vi "uBroker_Core.vi"(10 "ActorCore Transport":refnum<class "uTransport_uActor.lvclass">, 11 "brokerage queue in":refnum<queue>) -> (3 "brokerage queue out":refnum<queue>)   [LabVIEW 2021, in "uFramework.lvlib" / "uBroker.lvclass"]
doc: "This is a helper loop for the actor core. It reduces dynamic dispatching in the brokerage functions as it avoid contiuous recalls of the EXEC method."
uses:
  uBroker.lvclass
  uBroker.lvclass/uBroker.ctl
  uClient_Subscriber/uClient_Subscriber.lvclass
  Bin/uData.lvlibp/uData.lvclass
  <vilib>/Utility/miscctls.llb/LVMapReplaceAction.ctl
  uClient_Publisher/uClient_Publisher.lvclass
  uSubscription/uSubscription.lvclass
  uMsg/uMsg.lvclass
  uTransport_uActor/uTransport_uActor.lvclass
  TypeDef_uBrokerTopic.ctl
panel:
  in  "Subscribers":set{refnum<class "uClient_Subscriber.lvclass">}(c389)
  in  "Topics":map{string, T1}(c390)
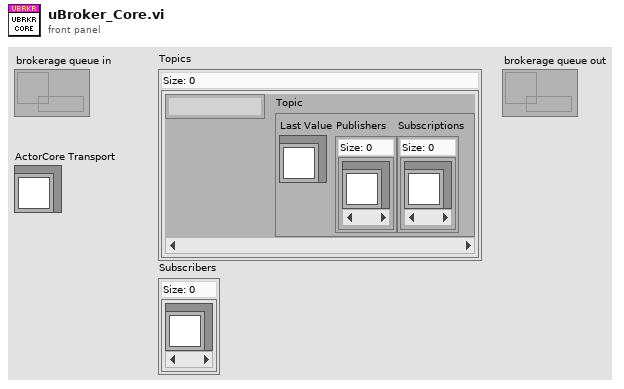
[diagram p1: front panel]
types:
  T1 = typedef "uFramework.lvlib/uBroker.lvclass/TypeDef_uBrokerTopic.ctl" = cluster{"Last Value":refnum<class "uMsg.lvclass">, "Publishers":set{refnum<class "uClient_Publisher.lvclass">}, "Subscriptions":set{refnum<class "uSubscription.lvclass">}}
  T2 = cluster{"Topics":map{string, T1}, "Subscribers":set{refnum<class "uClient_Subscriber.lvclass">}}
  T3 = typedef "LVMapReplaceAction.ctl" = enum32{"Modify Entry only if found", "Add or Modify Entry", "Delete Entry"}
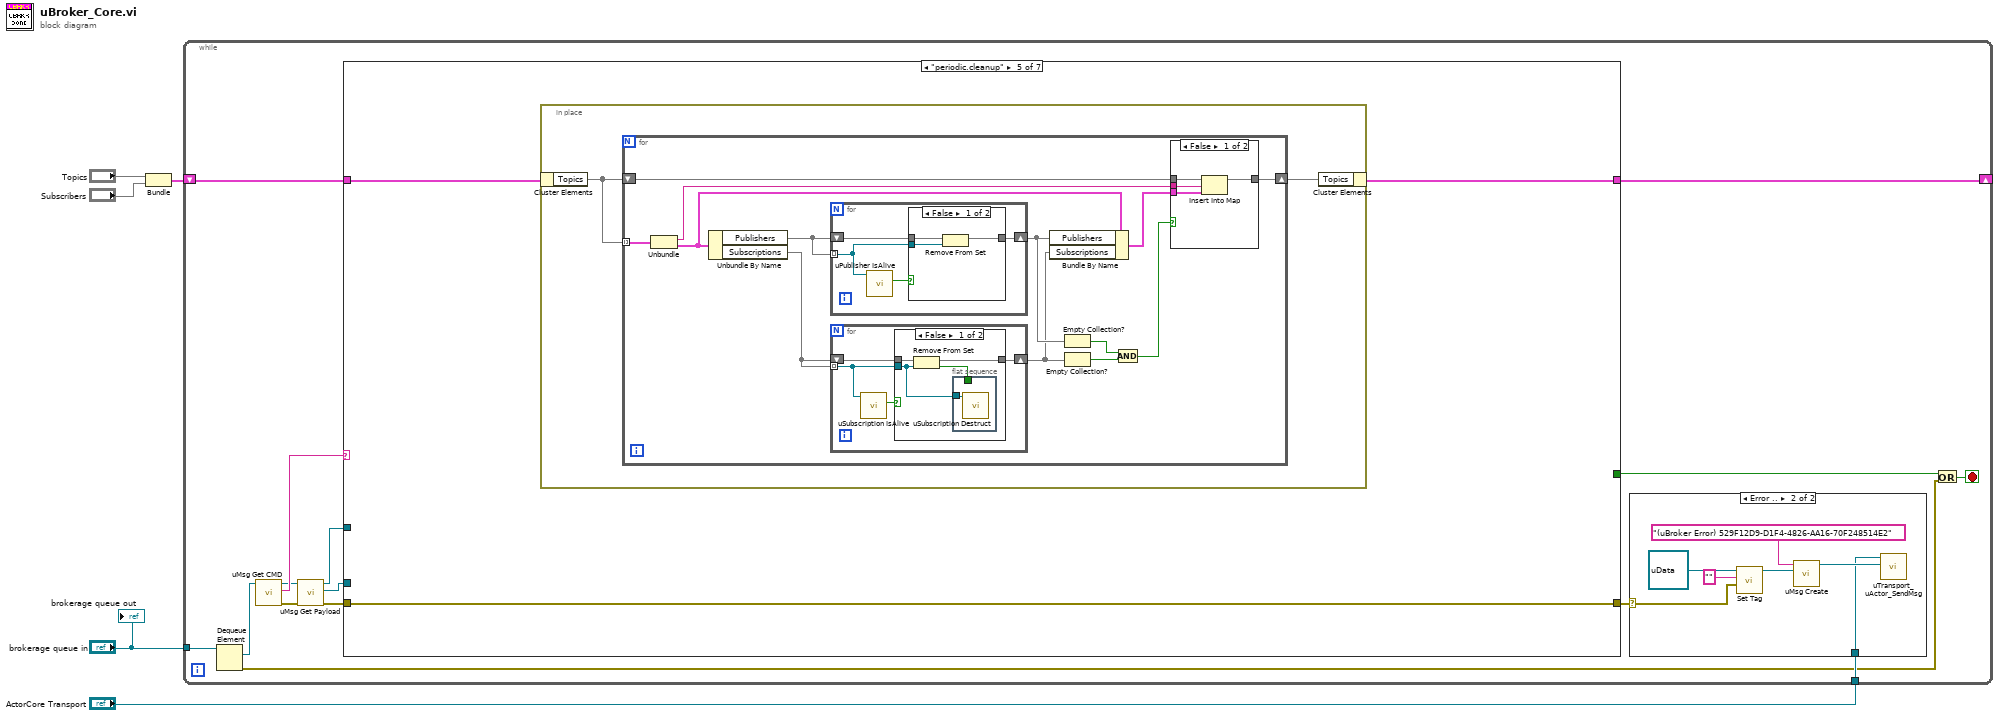
[diagram p0: block diagram]
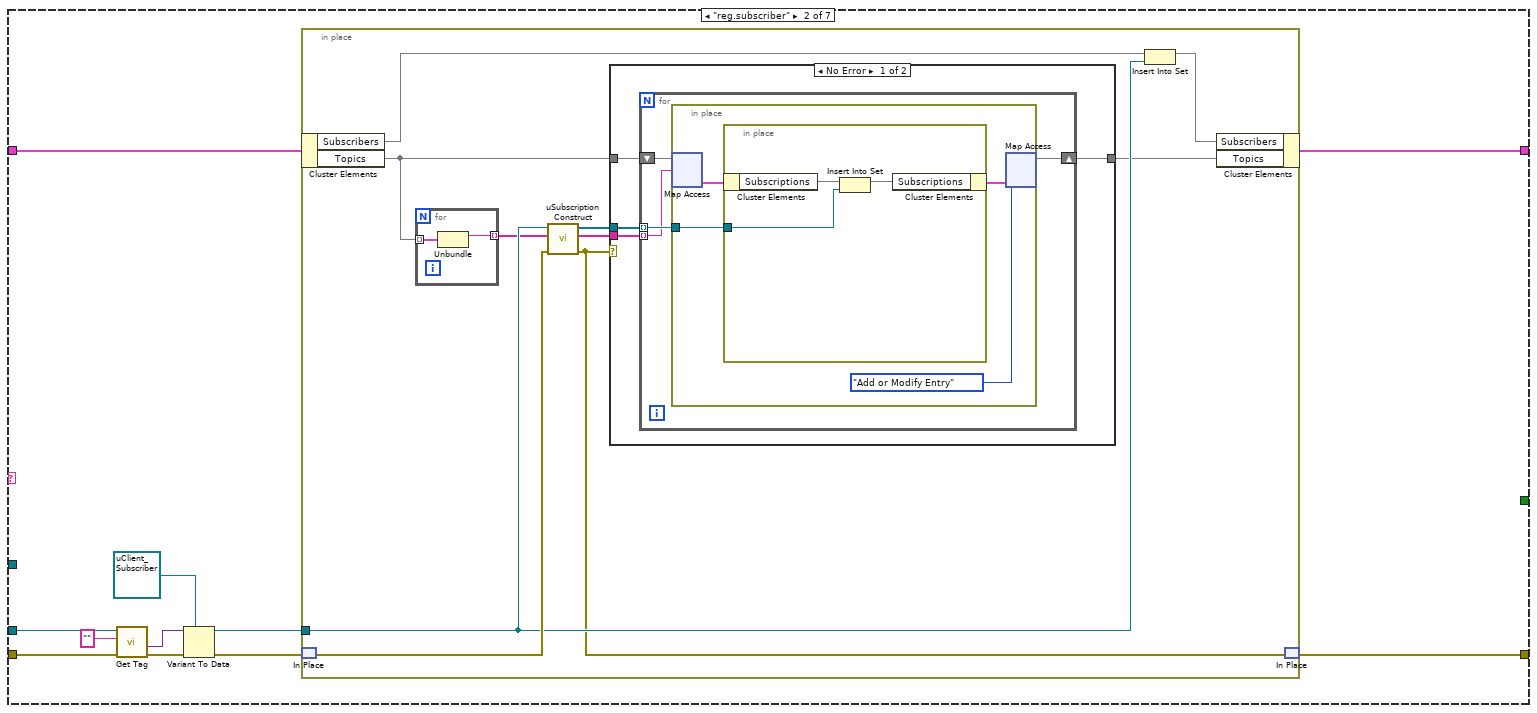
[diagram p4: hidden frame]
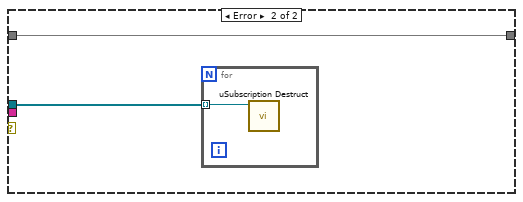
[diagram p5: hidden frame]
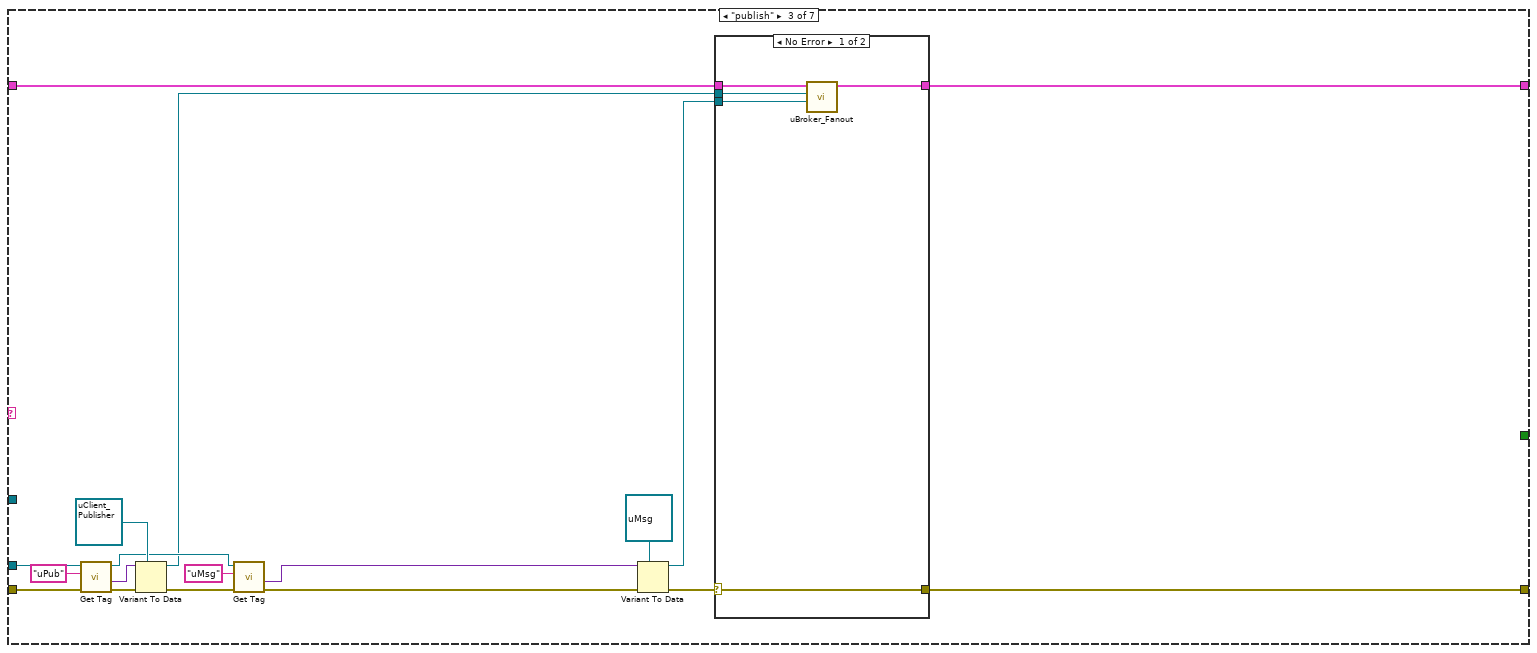
[diagram p6: hidden frame]
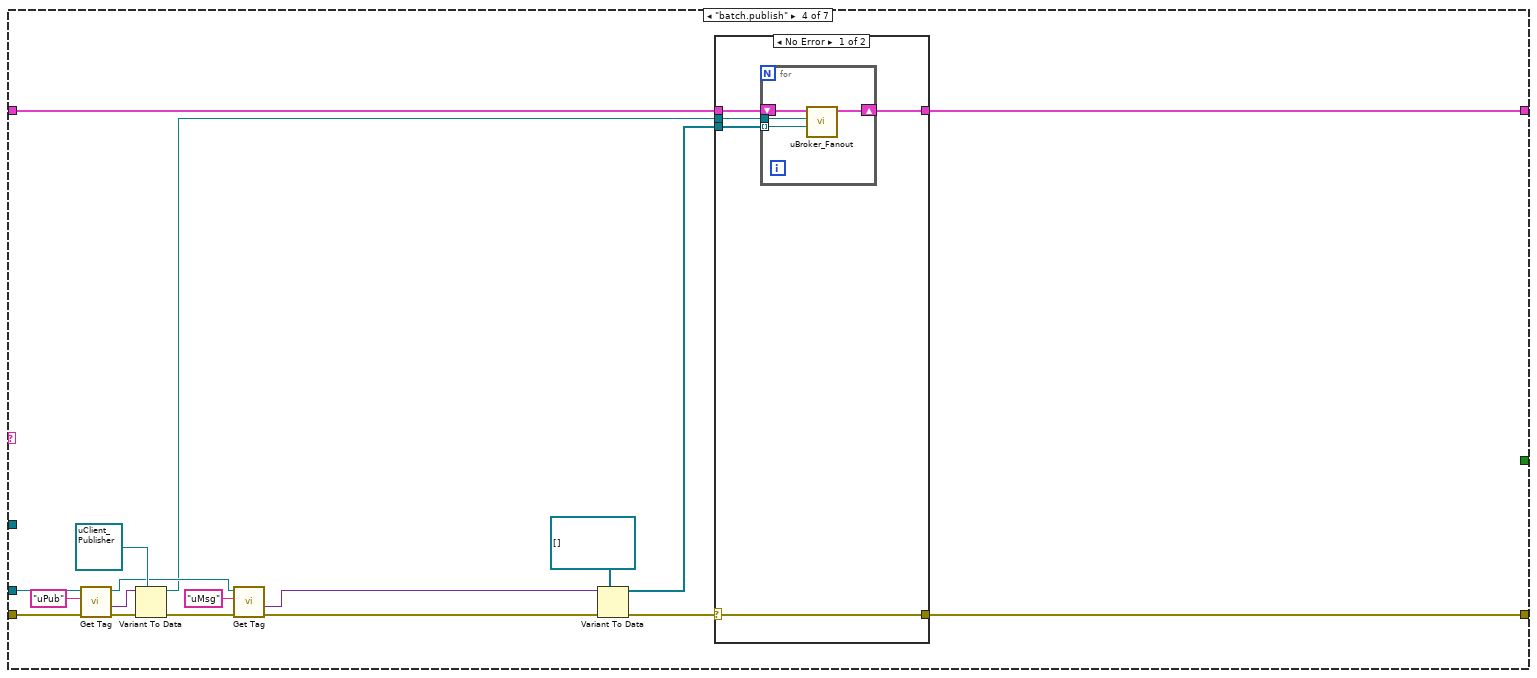
[diagram p8: hidden frame]
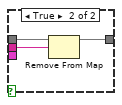
[diagram p10: hidden frame]
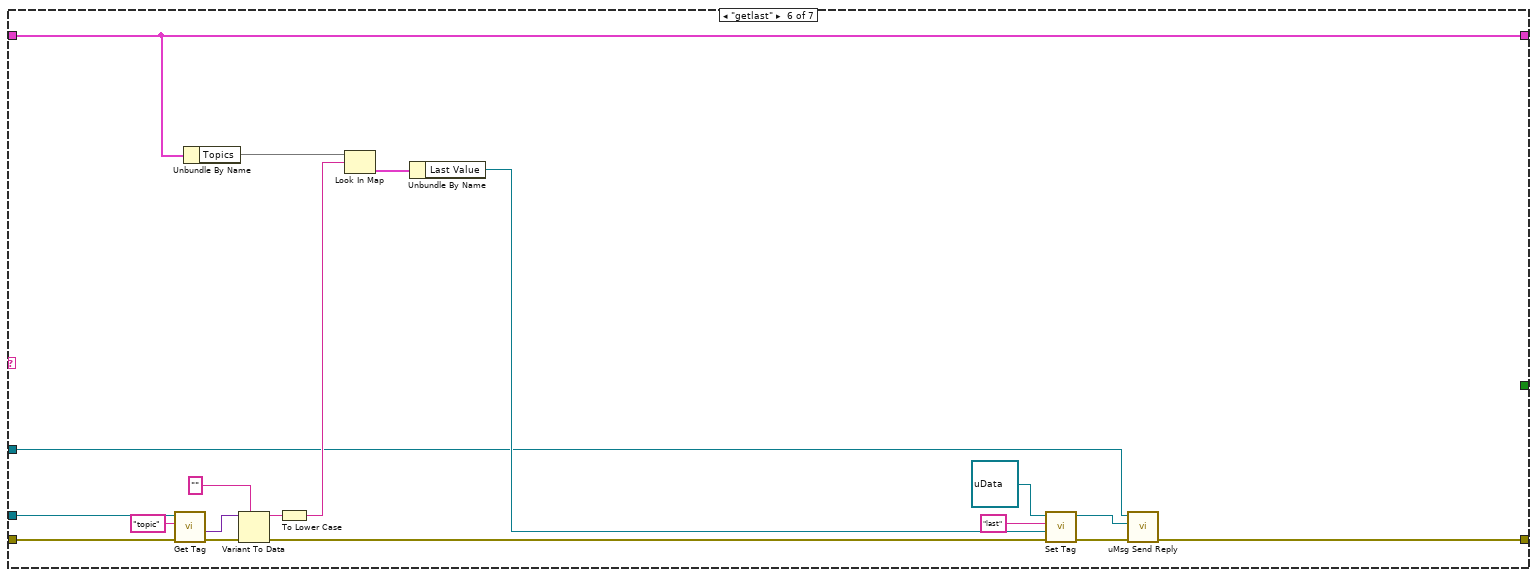
[diagram p13: hidden frame]
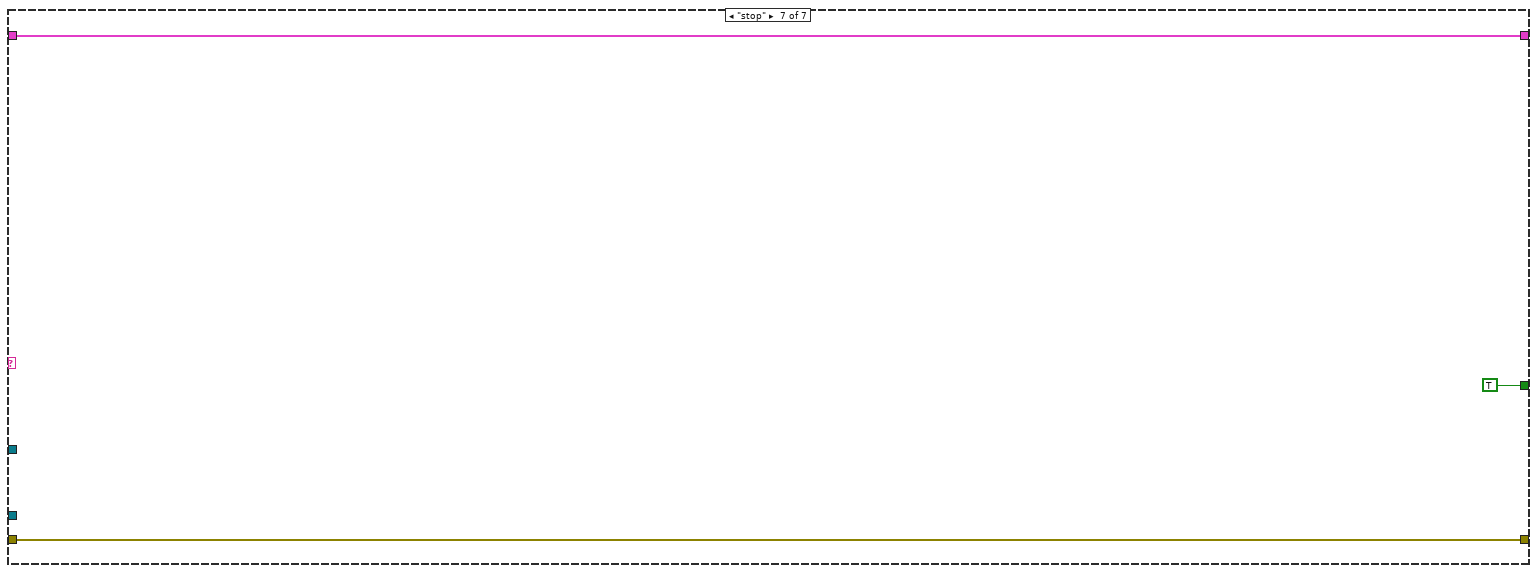
[diagram p14: hidden frame]
diagram:
  n1 = Bundle("Topics"="Topics", "Subscribers"="Subscribers") -> (w3:T2)  [unwired: 1 in]
  n2 = while {
    tunnel: "brokerage queue in" -> [w20]
    tunnel: "ActorCore Transport" -> [w16]
    shift-right: [w14] -> _
    shift-left: w3 -> [w15]
    stop <- w7 stop-if-true
    n3 = Dequeue Element(queue=w20) -> (element=w19:refnum<class "uMsg.lvclass">, error out=w8:errorcluster)  [unwired: 2 in, 2 out]
    n4 = call "uMsg Get CMD.vi"("uMsg in"=w19) -> ("error out"=w13:errorcluster, "CMD"=w18:string, "uMsg out"=w11:refnum<class "uMsg.lvclass">)  [unwired: 8 in]
    n5 = call "uMsg Get Payload.vi"("error in (no error)"=w13, "uMsg in"=w11) -> ("error out"=w12:errorcluster, "uData"=w10:refnum<class "uData.lvclass">, "uMsg out"=w6:refnum<class "uMsg.lvclass">)  [unwired: 7 in]
    n6 = case shown="\"periodic.cleanup\"" w18 {
      tunnel: w12 -> [w29 w33 w85 w110 w127 w184 w189]
      tunnel: [w29 w34 w76 w101 w127 w186 w189] -> w17
      tunnel: [w28 w30 w88 w113 w125 w185 w188] -> w14
      tunnel: w15 -> [w28 w31 w87 w112 w126 w185 w188]
      tunnel: w10 -> [_ w32 w86 w111 _ w183 _]
      tunnel: [_ _ _ _ _ _ TRUE] -> w9
      tunnel: w6 -> [_ _ _ _ _ w170 _]
      frame Default {
      }
      frame "reg.subscriber" {
        n7 = call "Get Tag.vi"("error in (no error)"=w33, "tag (case insensitive)"="", "uData in"=w32) -> ("error out"=w39:errorcluster, "value"=w38:variant)  [unwired: 5 in, 2 out]
        n8 = Variant To Data(error in=w39, type=refnum<class "uClient_Subscriber.lvclass"> refnum ("uSubscriber"), Variant=w38) -> (data=w36:refnum<class "uClient_Subscriber.lvclass">, error out=w35:errorcluster)
        n9 = in-place {
          in-place-border: w36 -> [w47]
          n10 = in-place-cluster #1(w31) -> ("Subscribers"=w49:set{refnum<class "uClient_Subscriber.lvclass">}, "Topics"=w45:map{string, T1})
          n11 = in-place-match #2(w35) -> (w50:errorcluster)
          n12 = for {
            tunnel: w45 -> [w70] mode=indexing
            tunnel: [w69] -> w46 mode=indexing
            n13 = Unbundle(w70) -> (w69:string)  [unwired: 1 out]
          }
          n14 = call "uSubscription Construct.vi"("error in (no error)"=w50, "Topics"=w46, "uClient_Subscriber"=w47) -> ("error out"=w43:errorcluster, "Filtered Topics"=w41:string[], "uSubscriptions out"=w44:refnum<class "uSubscription.lvclass">[])  [unwired: 6 in]
          n15 = case shown="No Error" w43 {
            tunnel: w45 -> [w54 w67]
            tunnel: w44 -> [w53 w66]
            tunnel: [w52 w67] -> w42
            tunnel: w41 -> [w51 _]
            frame No Error {
              n16 = for {
                tunnel: w53 -> [w57] mode=indexing
                shift-right: [w56] -> w52
                shift-left: w54 -> [w58]
                tunnel: w51 -> [w55] mode=indexing
                n17 = in-place {
                  in-place-border: w57 -> [w59]
                  n18 = in-place-map #3(w58, w55) -> (w61:T1)  [unwired: 1 in, 1 out]
                  n19 = in-place {
                    in-place-border: w59 -> [w63]
                    n20 = in-place-cluster #4(w61) -> ("Subscriptions"=w65:set{refnum<class "uSubscription.lvclass">})
                    n21 = Insert Into Set(10:w63, 11:w65) -> (3:w64:set{refnum<class "uSubscription.lvclass">})  [unwired: 1 out]
                    n22 = in-place-cluster #4("Subscriptions"=w64) -> (w60:T1)
                  }
                  n23 = in-place-map #3(w60, LVMapReplaceAction."Add or Modify Entry" ("action")) -> (w56:map{string, T1})  [unwired: 2 out]
                }
              }
            }
            frame Error {
              n24 = for {
                tunnel: w66 -> [w68] mode=indexing
                n25 = call "uSubscription Destruct.vi"("uSubscription in"=w68) -> ()  [unwired: 10 in, 1 out]
              }
            }
          }
          n26 = Insert Into Set(10:w47, 11:w49) -> (3:w48:set{refnum<class "uClient_Subscriber.lvclass">})  [unwired: 1 out]
          n27 = in-place-cluster #1("Subscribers"=w48, "Topics"=w42) -> (w30:T2)
          n28 = in-place-match #2(w43) -> (w34:errorcluster)
        }
      }
      frame "publish" {
        n29 = call "Get Tag.vi"("error in (no error)"=w85, "tag (case insensitive)"="uPub" ("uPublisher Tag"), "uData in"=w86) -> ("error out"=w83:errorcluster, "value"=w74:variant, "uData out"=w79:refnum<class "uData.lvclass">)  [unwired: 5 in, 1 out]
        n30 = Variant To Data(error in=w83, type=refnum<class "uClient_Publisher.lvclass"> refnum, Variant=w74) -> (data=w75:refnum<class "uClient_Publisher.lvclass">, error out=w81:errorcluster)
        n31 = call "Get Tag.vi"("error in (no error)"=w81, "tag (case insensitive)"="uMsg" ("uPublisher Tag"), "uData in"=w79) -> ("error out"=w78:errorcluster, "value"=w77:variant)  [unwired: 5 in, 2 out]
        n32 = Variant To Data(error in=w78, type=refnum<class "uMsg.lvclass"> refnum, Variant=w77) -> (data=w72:refnum<class "uMsg.lvclass">, error out=w73:errorcluster)
        n33 = case shown="No Error" w73 {
          selector: w73 -> [w93 w95]
          tunnel: w87 -> [w92 w94]
          tunnel: [w91 w94] -> w88
          tunnel: w72 -> [w89 _]
          tunnel: [w93 w95] -> w76
          tunnel: w75 -> [w90 _]
          frame No Error {
            n34 = call "uBroker_Fanout.vi"("uMsg"=w89, "uPub"=w90, "Cluster in"=w92) -> ("Cluster out"=w91:T2)  [unwired: 8 in]
          }
          frame Error {
          }
        }
      }
      frame "batch.publish" {
        n35 = call "Get Tag.vi"("error in (no error)"=w110, "tag (case insensitive)"="uPub" ("uPublisher Tag"), "uData in"=w111) -> ("error out"=w108:errorcluster, "value"=w99:variant, "uData out"=w104:refnum<class "uData.lvclass">)  [unwired: 5 in, 1 out]
        n36 = Variant To Data(error in=w108, type=refnum<class "uClient_Publisher.lvclass"> refnum, Variant=w99) -> (data=w100:refnum<class "uClient_Publisher.lvclass">, error out=w106:errorcluster)
        n37 = call "Get Tag.vi"("error in (no error)"=w106, "tag (case insensitive)"="uMsg" ("uPublisher Tag"), "uData in"=w104) -> ("error out"=w103:errorcluster, "value"=w102:variant)  [unwired: 5 in, 2 out]
        n38 = Variant To Data(error in=w103, type=refnum<class "uMsg.lvclass">[] [], Variant=w102) -> (data=w97:refnum<class "uMsg.lvclass">[], error out=w98:errorcluster)
        n39 = case shown="No Error" w98 {
          selector: w98 -> [w118 w124]
          tunnel: w112 -> [w117 w123]
          tunnel: [w116 w123] -> w113
          tunnel: w97 -> [w114 _]
          tunnel: [w118 w124] -> w101
          tunnel: w100 -> [w115 _]
          frame No Error {
            n40 = for {
              tunnel: w115 -> [w120]
              tunnel: w114 -> [w119] mode=indexing
              shift-right: [w121] -> w116
              shift-left: w117 -> [w122]
              n41 = call "uBroker_Fanout.vi"("uMsg"=w119, "uPub"=w120, "Cluster in"=w122) -> ("Cluster out"=w121:T2)  [unwired: 8 in]
            }
          }
          frame Error {
          }
        }
      }
      frame "periodic.cleanup" {
        n42 = in-place {
          n43 = in-place-cluster #5(w126) -> ("Topics"=w128:map{string, T1})
          n44 = for {
            tunnel: w128 -> [w140] mode=indexing
            shift-right: [w137] -> w129
            shift-left: w128 -> [w138]
            n45 = Unbundle(w140) -> (w135:string, "Topic"=w139:T1)
            n46 = Unbundle By Name(w139) -> ("Publishers"=w142:set{refnum<class "uClient_Publisher.lvclass">}, "Subscriptions"=w141:set{refnum<class "uSubscription.lvclass">})
            n47 = for {
              tunnel: w142 -> [w160] mode=indexing
              shift-right: [w162] -> w134
              shift-left: w142 -> [w163]
              n48 = call "uPublisher IsAlive.vi"("uClient_Publisher in"=w160) -> ("Is Alive?"=w161:bool)  [unwired: 8 in, 2 out]
              n49 = case shown="False" w161 {
                tunnel: w163 -> [w166 w167]
                tunnel: [w165 w167] -> w162
                tunnel: w160 -> [w164 _]
                frame False {
                  n50 = Remove From Set(10:w164, 11:w166) -> (3:w165:set{refnum<class "uClient_Publisher.lvclass">})  [unwired: 1 out]
                }
                frame True {
                }
              }
            }
            n51 = for {
              tunnel: w141 -> [w150] mode=indexing
              shift-right: [w152] -> w133
              shift-left: w141 -> [w153]
              n52 = call "uSubscription IsAlive.vi"("uSubscription in"=w150) -> ("Is Alive?"=w151:bool)  [unwired: 9 in, 1 out]
              n53 = case shown="False" w151 {
                tunnel: w153 -> [w157 w159]
                tunnel: [w156 w159] -> w152
                tunnel: w150 -> [w155 _]
                frame False {
                  n54 = Remove From Set(10:w155, 11:w157) -> (2:w154:bool, 3:w156:set{refnum<class "uSubscription.lvclass">})
                  n55 = flat-sequence {
                    tunnel: w155 -> [w158]
                    tunnel: w154 -> [_]
                    frame #0 {
                      n56 = call "uSubscription Destruct.vi"("uSubscription in"=w158) -> ()  [unwired: 10 in, 1 out]
                    }
                  }
                }
                frame True {
                }
              }
            }
            n57 = Bundle By Name(cluster=w139, "Publishers"=w134, "Subscriptions"=w133) -> (w136:T1)
            n58 = Empty Collection?(1:w134) -> (0:w131:bool)
            n59 = Empty Collection?(1:w133) -> (0:w132:bool)
            n60 = And(x=w131, y=w132) -> (x .and. y?=w130:bool)
            n61 = case shown="False" w130 {
              tunnel: w138 -> [w146 w149]
              tunnel: [w145 w148] -> w137
              tunnel: w136 -> [w144 _]
              tunnel: w135 -> [w143 w147]
              frame False {
                n62 = Insert Into Map(map in=w146, key=w143, value=w144) -> (map out=w145:map{string, T1})  [unwired: 2 out]
              }
              frame True {
                n63 = Remove From Map(10:w147, 11:w149) -> (3:w148:map{string, T1})  [unwired: 2 out]
              }
            }
          }
          n64 = in-place-cluster #5("Topics"=w129) -> (w125:T2)
        }
      }
      frame "getlast" {
        n65 = call "Get Tag.vi"("error in (no error)"=w184, "tag (case insensitive)"="topic", "uData in"=w183) -> ("error out"=w181:errorcluster, "value"=w180:variant)  [unwired: 5 in, 2 out]
        n66 = Unbundle By Name(w185) -> ("Topics"=w168:map{string, T1})
        n67 = Variant To Data(error in=w181, type="" ("tag (case insensitive)"), Variant=w180) -> (data=w179:string, error out=w175:errorcluster)
        n68 = To Lower Case(string=w179) -> (all lower case string=w177:string)
        n69 = Look In Map(map=w168, key=w177) -> (value=w176:T1)  [unwired: 1 in, 1 out]
        n70 = Unbundle By Name(w176) -> ("Last Value"=w173:refnum<class "uMsg.lvclass">)
        n71 = call "Set Tag.vi"("error in (no error)"=w175, "Variant"=w173, "tag (case insensitive)"="last", "uData in"=refnum<class "uData.lvclass"> refnum) -> ("error out"=w169:errorcluster, "uData out"=w171:refnum<class "uData.lvclass">)  [unwired: 5 in, 1 out]
        n72 = call "uMsg Send Reply.vi"("error in (no error)"=w169, "Reply Data"=w171, "Original Msg"=w170) -> ("error out"=w186:errorcluster)  [unwired: 8 in]
      }
      frame "stop" {
      }
    }
    n73 = case shown="Error .." w17 {
      selector: w17 -> [_ w24]
      tunnel: w16 -> [_ w21]
      frame No Error {
      }
      frame Error {
        n74 = call "Set Tag.vi"("Variant"=w24, "tag (case insensitive)"="", "uData in"=refnum<class "uData.lvclass"> refnum) -> ("uData out"=w26:refnum<class "uData.lvclass">)  [unwired: 6 in, 2 out]
        n75 = call "uMsg Create.vi"("Payload"=w26, "CMD"="(uBroker Error) 529F12D9-D1F4-4826-AA16-70F248514E2") -> ("uMsg out"=w22:refnum<class "uMsg.lvclass">)  [unwired: 8 in, 1 out]
        n76 = call "uTransport_uActor_SendMsg.vi"("Msg"=w22, "uTransport_uActor in"=w21) -> ()  [unwired: 9 in, 1 out]
      }
    }
    n77 = Or(x=w9, y=w8) -> (x .or. y?=w7:bool)
  }
  "brokerage queue out" <- "brokerage queue in"
